vi "弹窗-设置周期.vi"() -> ()   [LabVIEW 2017]
panel:
  out "参考-单位":enum16{"年", "月", "日", "时", "分"}(ring)
  out "参考-定时模式":enum16{"绝对时间", "相对时间"}(ring)
  in  "超时":i32=1000
  out "目标时刻-导出":timestamp
  out "目标时刻-累积":timestamp
  out "定时器":T1
  in  "分别导出?":bool
  out "下个导出时刻":string
  in  "间隔-导出":u8=1 min=1 max=23
  in  "单位-导出":enum16{"年", "月", "日", "时", "分"}(ring)=enum."日"
  in  "定时模式-导出":enum16{"绝对时间", "相对时间"}(ring)
  out "提示语":string
  out "下个累积时刻":string caption="下个导出时刻"
  in  "间隔-累积":u8=1 min=1 max=59
  in  "单位-累积":enum16{"年", "月", "日", "时", "分"}(ring)=enum."日"
  in  "定时模式-累积":enum16{"绝对时间", "相对时间"}(ring)
  in  "确定":bool
  in  "取消":bool
  out "信号-关闭窗口":bool=TRUE
  # "累积周期"
  # "导出周期"
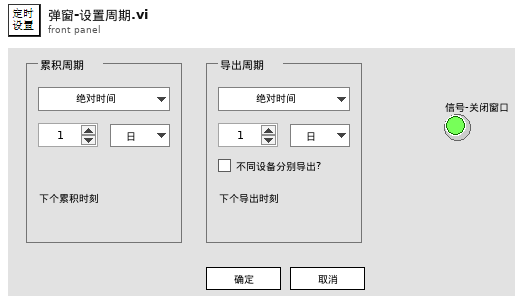
[diagram p1: front panel]
types:
  T1 = typedef "定时器枚举.ctl" = enum16{"累积定时", "导出定时"}
  T2 = typedef "定时配置.ctl" = cluster{"定时模式":enum16{"绝对时间", "相对时间"}, "单位":enum16{"年", "月", "日", "时", "分"}, "间隔":u8, "目标时刻":timestamp}
  T3 = enum32{"Invalid", "Standard", "Closed", "Hidden", "Minimized", "Maximized"}
  T4 = typedef "簇-输入.ctl" = cluster{"配置文件动作":T5, "数据输入":variant}
  T5 = typedef "枚举-配置文件动作.ctl" = enum16{"初始化加载配置", "读取配置", "写入-屏幕键盘", "写入-静音延迟", "写入-主要探头类型", "写入-串口配置", "写入-累积定时", "写入-导出定时", "保存配置到文件"}
  T6 = typedef "簇-定时配置.ctl" = cluster{"定时模式":enum16{"绝对时间", "相对时间"}, "单位":enum16{"年", "月", "日", "时", "分"}, "间隔":u8, "目标时刻":timestamp}
  T7 = typedef "簇-配置文件内容.ctl" = cluster{"调试模式？":bool, "屏幕键盘？":bool, "软件版本":string, "静音延迟 s":u16, "主要探头类型":T8, "串口配置":cluster{"COM口":refnum<visa-resource-name>, "波特率":enum16{"9600", "19200"}, "读写超时ms":i16, "丢包判定次数":i16}, "定时配置-累积分段":T6, "定时配置-自动导出":cluster{"定时配置-自动导出":T6, "分别导出?":bool}}
  T8 = typedef "枚举-主要探头类型.ctl" = enum16{"网络探头", "串口探头"}
  T9 = typedef "LVDateTimeRec.ctl" = cluster{"秒数的小数部分":dbl, "秒":i32, "分":i32, "时":i32, "日":i32, "月":i32, "年":i32, "天数（周）":i32, "天数（年）":i32, "DST":i32}
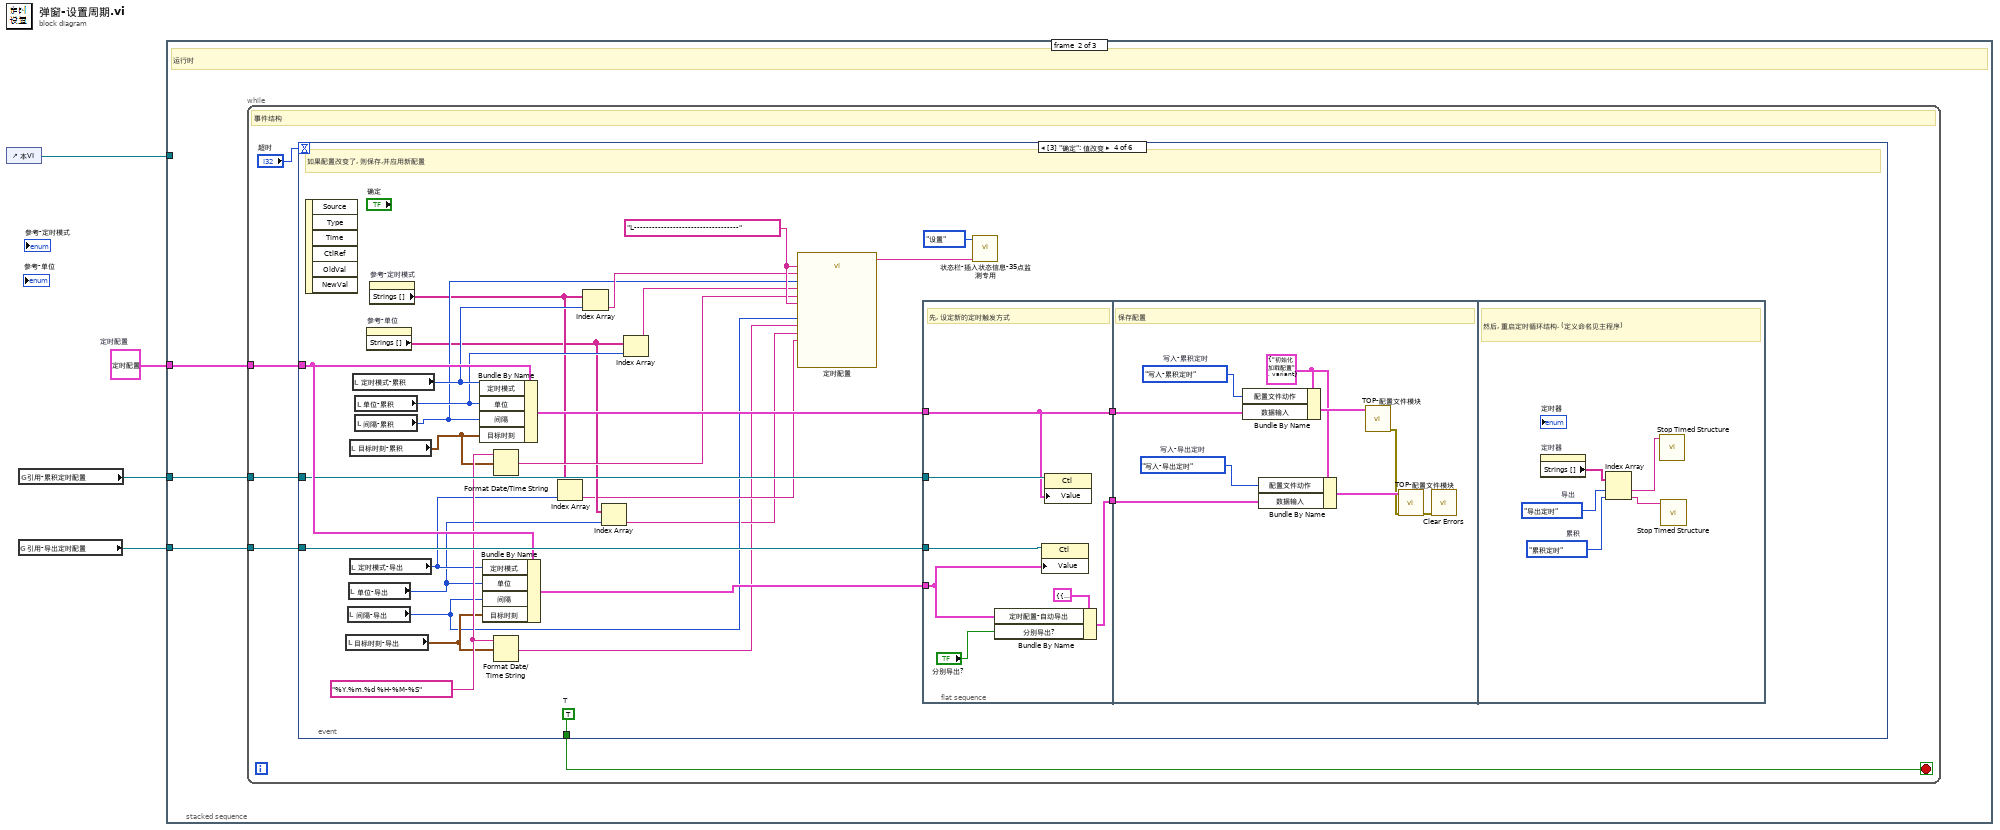
[diagram p0: block diagram]
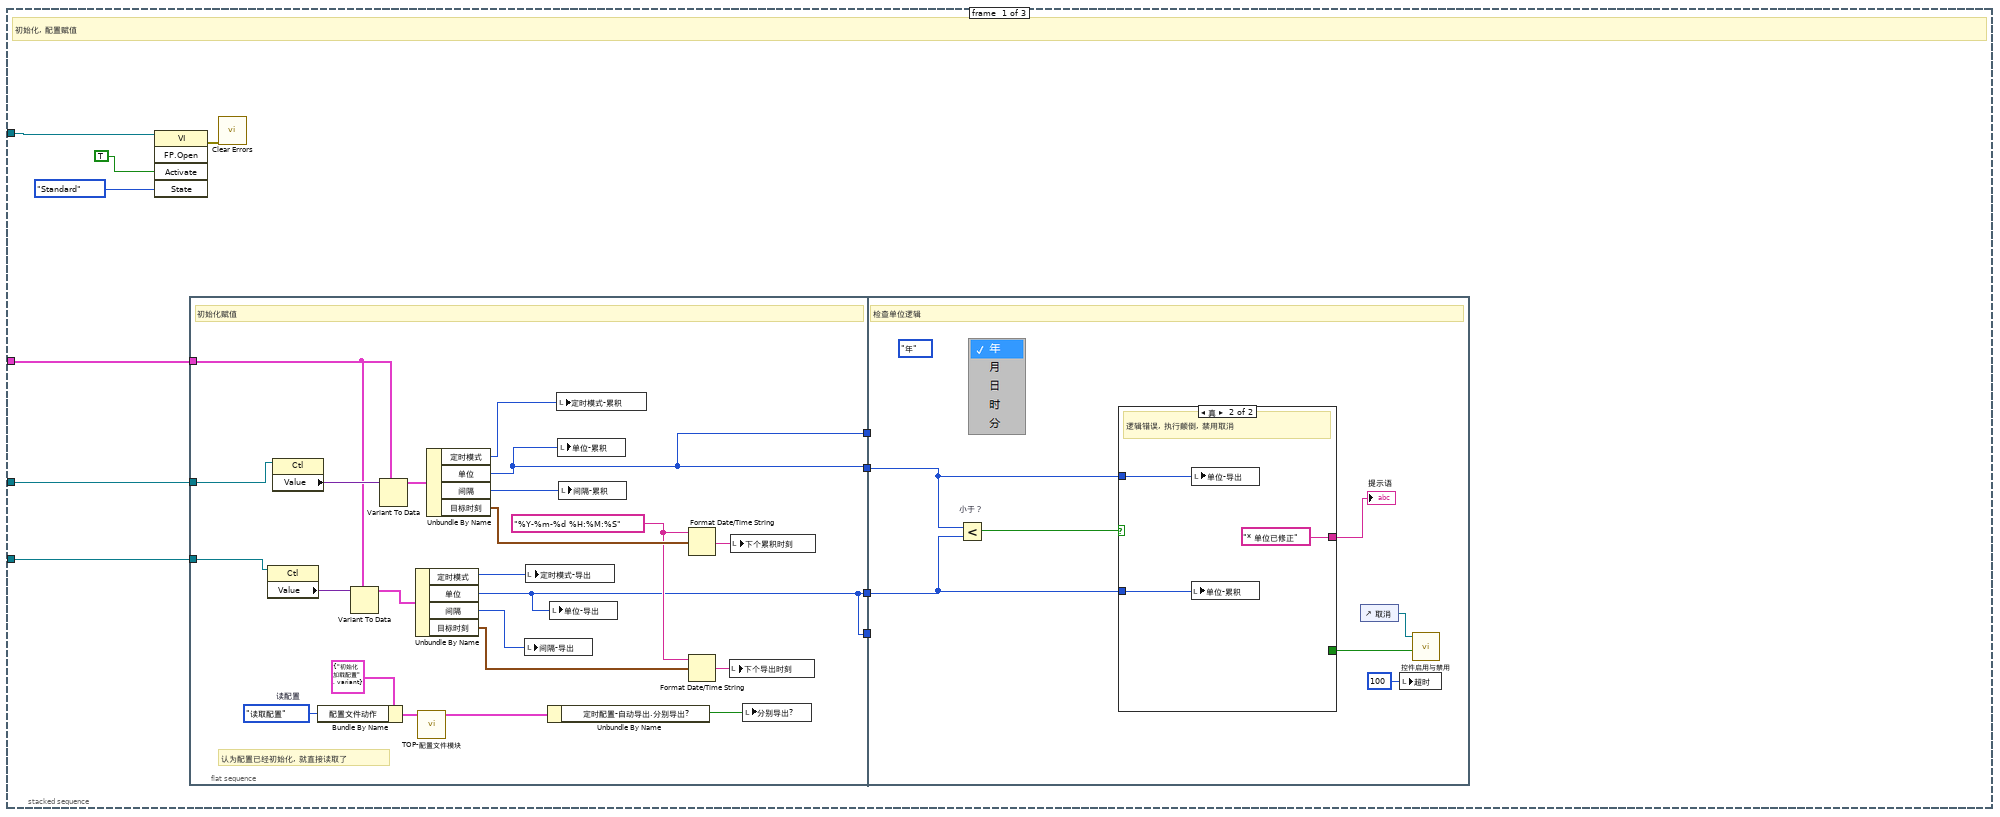
[diagram p2: hidden frame]
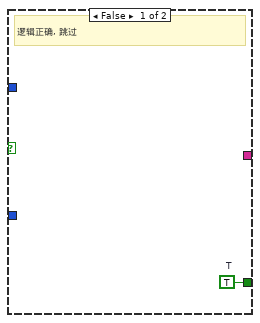
[diagram p3: hidden frame]
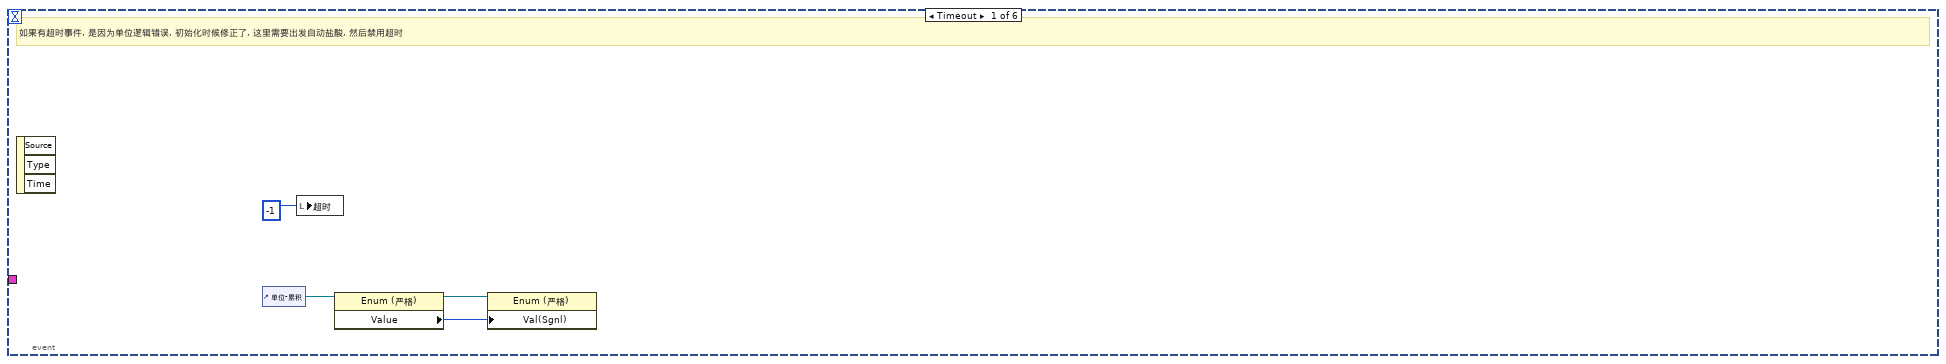
[diagram p4: hidden frame]
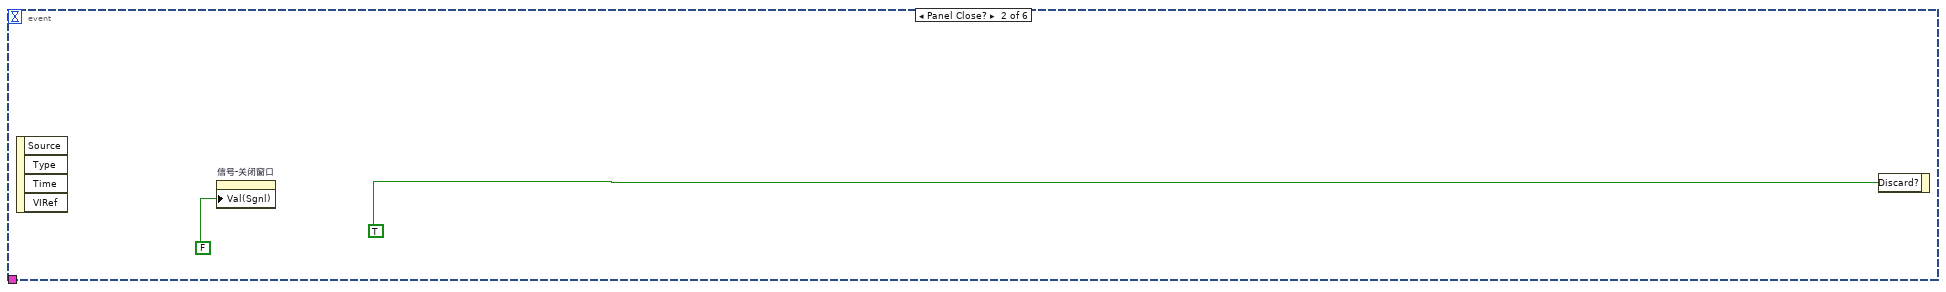
[diagram p5: hidden frame]
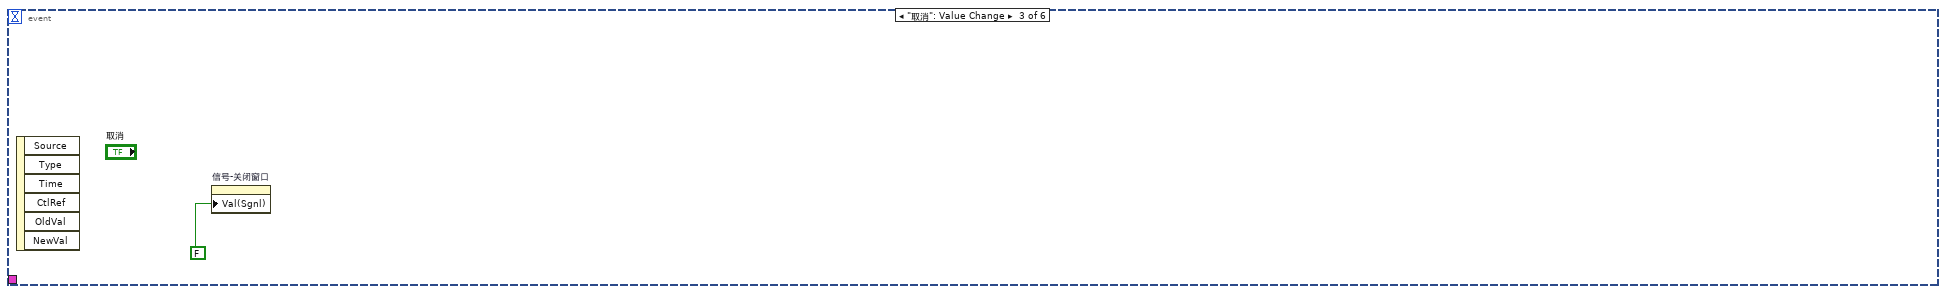
[diagram p6: hidden frame]
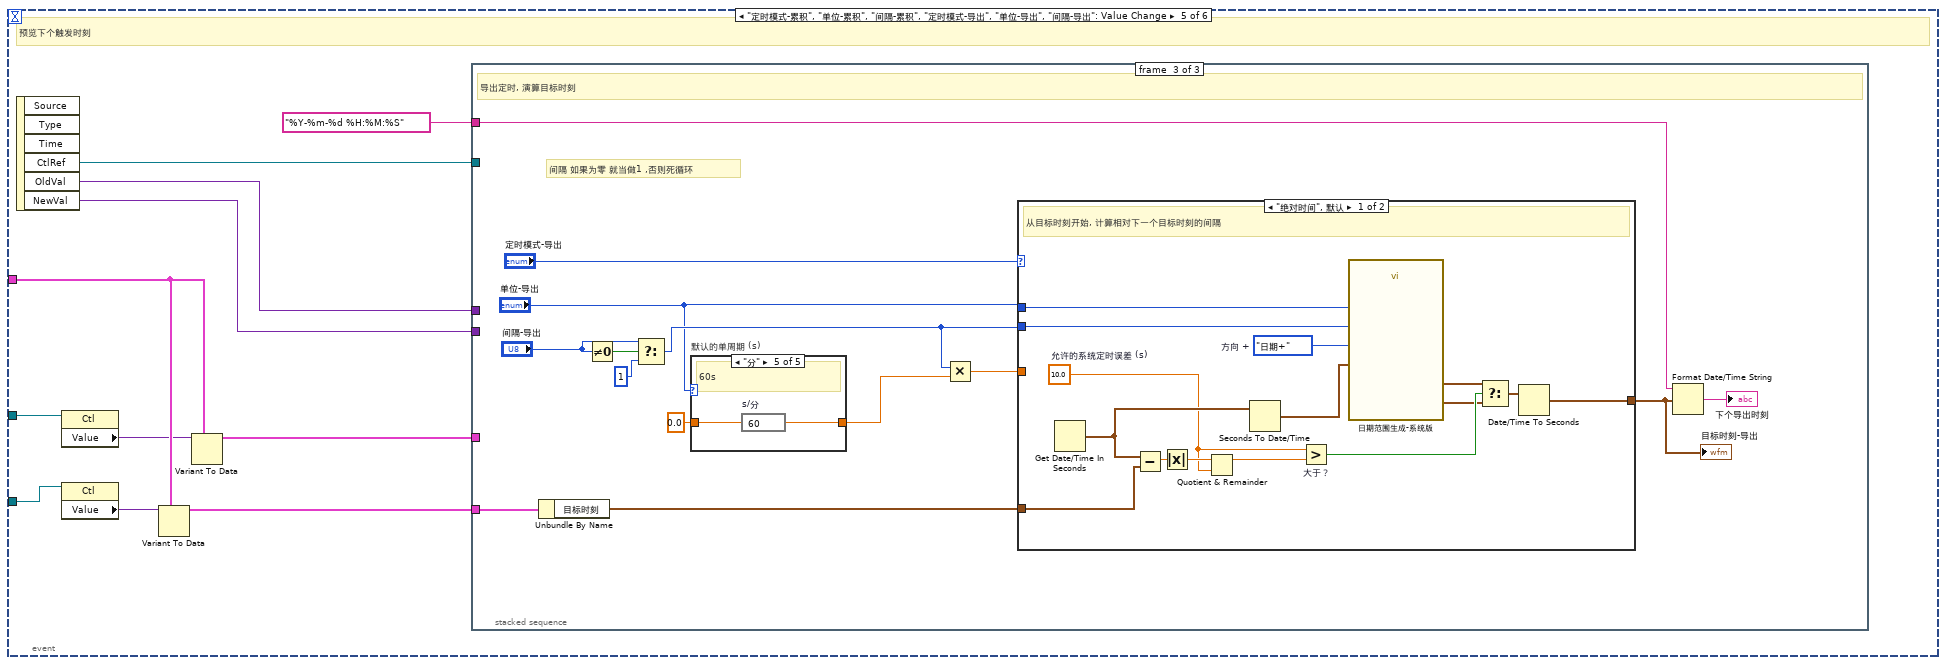
[diagram p7: hidden frame]
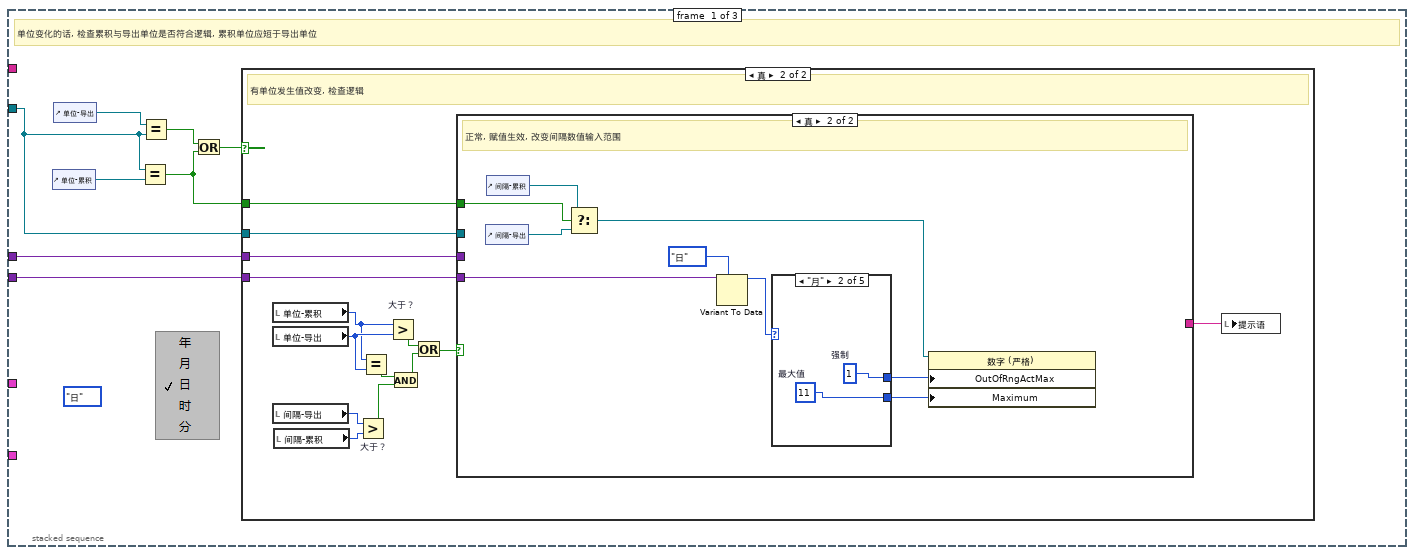
[diagram p8: hidden frame]
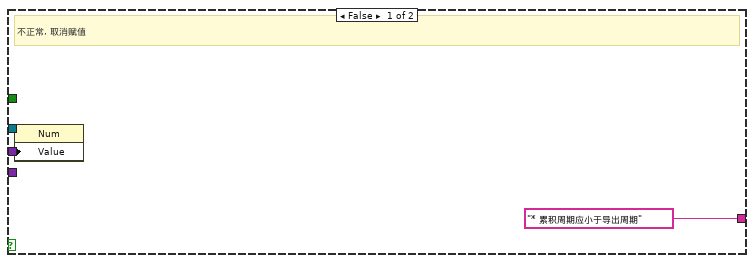
[diagram p10: hidden frame]
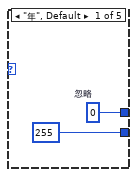
[diagram p11: hidden frame]
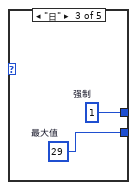
[diagram p12: hidden frame]
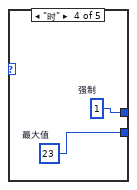
[diagram p13: hidden frame]
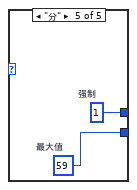
[diagram p14: hidden frame]
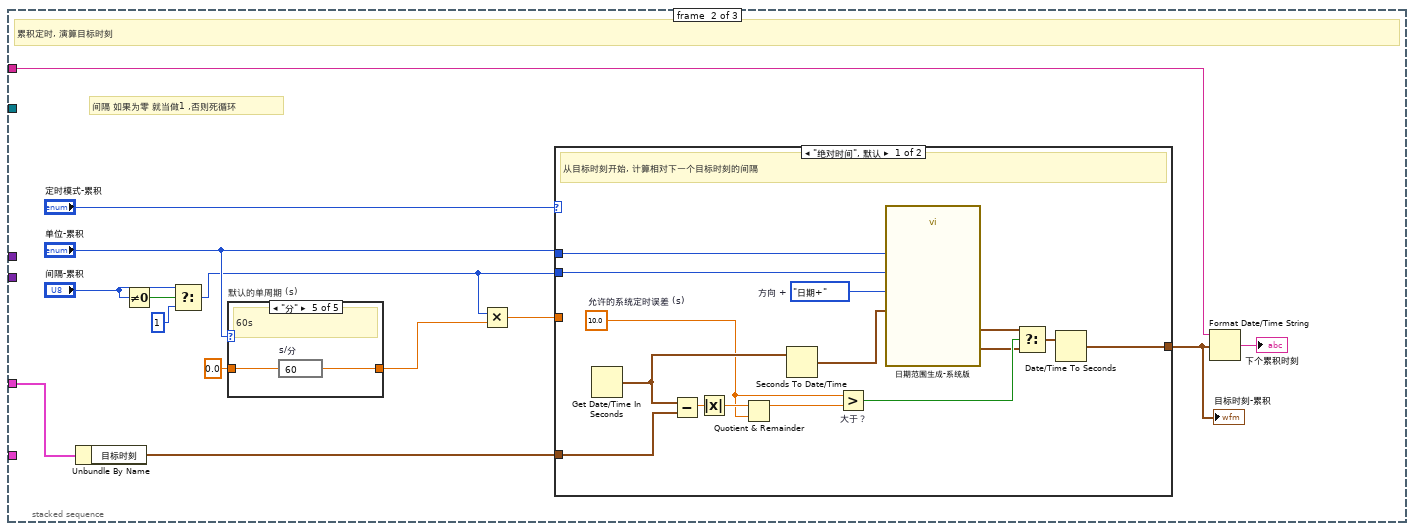
[diagram p15: hidden frame]
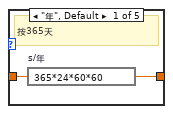
[diagram p16: hidden frame]
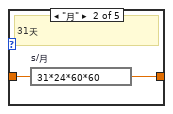
[diagram p17: hidden frame]
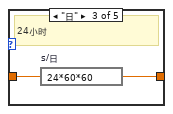
[diagram p18: hidden frame]
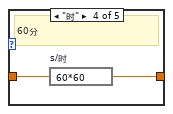
[diagram p19: hidden frame]
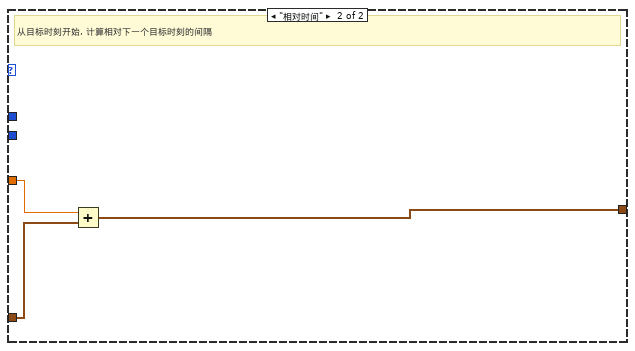
[diagram p20: hidden frame]
diagram:
  w3 = T2 {"定时模式"=enum."绝对时间", "单位"=enum."年", "间隔"=0, "目标时刻"=timestamp(0 s since 1904-01-01)}  # 定时配置
  n1 = control-ref of="本VI"() -> (w4:refnum<vi>)
  n2 = global read "全局变量-35点监测.vi" "引用-导出定时配置"() -> (w2:refnum<vi>)
  n3 = global read "全局变量-35点监测.vi" "引用-累积定时配置"() -> (w1:refnum<vi>)
  n4 = stacked-sequence {
    tunnel: w4 -> [w15 _ w257]
    tunnel: w2 -> [w11 w52 _]
    tunnel: w3 -> [w10 w51 _]
    tunnel: w1 -> [w12 w50 _]
    frame #0 {
      # "初始化, 配置赋值"
      n5 = invoke class="VI" method="FP.Open"(reference=w15, "Activate"=TRUE ("激活？"), "State"=T3."Standard" ("状态")) -> (error out=w9:errorcluster)  [unwired: 2 in, 4 out]
      n6 = flat-sequence {
        tunnel: w12 -> [w30]
        tunnel: w11 -> [w29]
        tunnel: w10 -> [w28]
        tunnel: [w21] -> w8
        tunnel: [w20] -> w7
        tunnel: [w21] -> w6
        tunnel: [w20] -> w5
        tunnel: w8 -> [w44]
        tunnel: w7 -> [w43]
        tunnel: w6 -> [_]
        tunnel: w5 -> [_]
        frame #0 {
          w16 = 枚举-配置文件动作."读取配置"  # 读配置
          w24 = "%Y-%m-%d %H:%M:%S" ("时间格式字符串(%c)")
          # "认为配置已经初始化, 就直接读取了"
          # "初始化赋值"
          n7 = property class="Ctl"(reference=w29) -> ("Value"=w32:variant)  [unwired: 1 in, 2 out]
          n8 = property class="Ctl"(reference=w30) -> ("Value"=w37:variant)  [unwired: 1 in, 2 out]
          n9 = Bundle By Name(cluster=T4 {"配置文件动作"=enum."初始化加载配置", "数据输入"=variant} ("输入"), "配置文件动作"=w16) -> (w17:T4)
          n10 = Variant To Data(type=w28, Variant=w32) -> (data=w31:T2)  [unwired: 1 in, 1 out]
          n11 = Variant To Data(type=w28, Variant=w37) -> (data=w38:T2)  [unwired: 1 in, 1 out]
          n12 = Unbundle By Name(w31) -> ("定时模式"=w26:enum16{"绝对时间", "相对时间"}, "单位"=w20:enum16{"年", "月", "日", "时", "分"}, "间隔"=w25:u8, "目标时刻"=w23:timestamp)
          n13 = call "TOP-配置文件模块.vi"("输入"=w17) -> ("配置文件"=w19:T7)  [unwired: 9 in, 1 out]
          n14 = Unbundle By Name(w38) -> ("定时模式"=w33:enum16{"绝对时间", "相对时间"}, "单位"=w21:enum16{"年", "月", "日", "时", "分"}, "间隔"=w34:u8, "目标时刻"=w36:timestamp)
          n15 = local write "间隔-导出"(w25) -> ()
          n16 = local write "定时模式-导出"(w26) -> ()
          n17 = Unbundle By Name(w19) -> ("定时配置-自动导出.分别导出?"=w27:bool)
          n18 = local write "单位-导出"(w20) -> ()
          n19 = local write "定时模式-累积"(w33) -> ()
          n20 = local write "单位-累积"(w21) -> ()
          n21 = local write "间隔-累积"(w34) -> ()
          n22 = Format Date/Time String(time format string (%c)=w24, seconds (now)=w36) -> (date/time string=w35:string)  [unwired: 1 in]
          n23 = Format Date/Time String(time format string (%c)=w24, seconds (now)=w23) -> (date/time string=w22:string)  [unwired: 1 in]
          n24 = local write "下个导出时刻"(w22) -> ()
          n25 = local write "下个累积时刻"(w35) -> ()
          n26 = local write "分别导出?"(w27) -> ()
        }
        frame #1 {
          (unwired) enum16{"年", "月", "日", "时", "分"}."年" ("单位")
          # "检查单位逻辑"
          n27 = Less? "小于？"(x=w44, y=w43) -> (x < y?=w45:bool)
          n28 = case shown="真" w45 {
            tunnel: w44 -> [_ w49]
            tunnel: w43 -> [_ w48]
            tunnel: [_ "* 单位已修正" ("提示语")] -> w40
            tunnel: [w46 _] -> w41
            frame False {
              w46 = TRUE  # T
              # "逻辑正确, 跳过"
            }
            frame True {
              # "逻辑错误, 执行颠倒, 禁用取消"
              n29 = local write "单位-累积"(w48) -> ()
              n30 = local write "单位-导出"(w49) -> ()
            }
          }
          "提示语" <- w40
          n31 = control-ref of="取消"() -> (w42:refnum<vi>)
          n32 = local write "超时"(100 ("超时")) -> ()
          n33 = call "控件启用与禁用.vi"("启用？"=w41, "控件引用"=w42) -> ()  [unwired: 9 in, 1 out]
        }
      }
      n34 = call <vilib>:"Clear Errors.vi"("error in (no error)"=w9) -> ()  [unwired: 5 in, 2 out]
    }
    frame #1 {
      # "运行时"
      n35 = while {
        tunnel: w52 -> [w56]
        tunnel: w51 -> [w55]
        tunnel: w50 -> [w54]
        stop <- w57 stop-if-true
        # "事件结构"
        n36 = event shown="[3] \"确定\": 值改变" {
          selector: _ -> [_ _ _ _ _ _]
          dyn-events: _ -> [_ _ _ _ _ _]
          timeout: "超时" -> [_ _ _ _ _ _]
          tunnel: [_ _ _ w92 _ TRUE] -> w57
          tunnel: w56 -> [_ _ _ w91 w123 _]
          tunnel: w55 -> [_ _ _ w88 w121 _]
          tunnel: w54 -> [_ _ _ w87 w122 _]
          event Timeout {
            # "如果有超时事件, 是因为单位逻辑错误, 初始化时候修正了, 这里需要出发自动盐酸, 然后禁用超时"
            n37 = event-data() -> ()  [unwired: 1 in, 3 out]
            n38 = control-ref of="单位-累积"() -> (w60:refnum<vi>)
            n39 = local write "超时"(-1 ("超时")) -> ()
            n40 = property class="Enum (严格)"(reference=w60) -> (reference out=w59:refnum<vi>, "Value"=w58:enum16{"年", "月", "日", "时", "分"})  [unwired: 1 in, 1 out]
            n41 = property class="Enum (严格)"(reference=w59, "Val(Sgnl)"=w58) -> ()  [unwired: 1 in, 2 out]
          }
          event Panel Close? {
            n42 = event-data() -> ()  [unwired: 1 in, 4 out]
            n43 = property on="信号-关闭窗口" class="Bool (严格)"("Val(Sgnl)"=FALSE ("值(信号)")) -> ()  [unwired: 2 in, 2 out]
            n44 = event-data("Discard?"=TRUE ("放弃？")) -> ()  [unwired: 1 in, 1 out]
          }
          event "取消": Value Change {
            n45 = event-data() -> ()  [unwired: 1 in, 6 out]
            n46 = property on="信号-关闭窗口" class="Bool (严格)"("Val(Sgnl)"=FALSE ("值(信号)")) -> ()  [unwired: 2 in, 2 out]
          }
          event "确定": Value Change {
            w80 = "%Y.%m.%d %H-%M-%S" ("时间格式字符串(%c)")
            w77 = "L-----------------------------------" ("字符串")
            w92 = TRUE  # T
            # "如果配置改变了, 则保存,并应用新配置"
            n47 = event-data() -> ()  [unwired: 1 in, 6 out]
            n48 = local read "目标时刻-导出"() -> (w79:timestamp)
            n49 = local read "间隔-导出"() -> (w67:u8)
            n50 = local read "单位-导出"() -> (w69:enum16{"年", "月", "日", "时", "分"})
            n51 = local read "目标时刻-累积"() -> (w78:timestamp)
            n52 = local read "定时模式-导出"() -> (w70:enum16{"绝对时间", "相对时间"})
            n53 = local read "定时模式-累积"() -> (w83:enum16{"绝对时间", "相对时间"})
            n54 = local read "单位-累积"() -> (w81:enum16{"年", "月", "日", "时", "分"})
            n55 = local read "间隔-累积"() -> (w75:u8)
            n56 = property on="参考-单位" class="Enum (严格)"() -> ("Strings []"=w71:string[])  [unwired: 2 in, 2 out]
            n57 = property on="参考-定时模式" class="Enum (严格)"() -> ("Strings []"=w72:string[])  [unwired: 2 in, 2 out]
            n58 = Bundle By Name(cluster=w88, "定时模式"=w83, "单位"=w81, "间隔"=w75, "目标时刻"=w78) -> (w90:T2)
            n59 = Bundle By Name(cluster=w88, "定时模式"=w70, "单位"=w69, "间隔"=w67, "目标时刻"=w79) -> (w86:T2)
            n60 = Format Date/Time String(time format string (%c)=w80, seconds (now)=w78) -> (date/time string=w73:string)  [unwired: 1 in]
            n61 = Format Date/Time String(time format string (%c)=w80, seconds (now)=w79) -> (date/time string=w65:string)  [unwired: 1 in]
            n62 = Index Array(array=w72, index=w70) -> (element=w68:string)
            n63 = Index Array(array=w72, index=w83) -> (element=w76:string)
            n64 = Index Array(array=w71, index=w69) -> (element=w66:string)
            n65 = Index Array(array=w71, index=w81) -> (element=w74:string)
            n66 = call "定时配置"("补充_累"=w77, "模式_累"=w76, "间隔_累"=w75, "周期_类"=w74, "下个_累"=w73, "补充_导"=w77, "模式_导"=w68, "间隔_导"=w67, "周期_导"=w66, "下个_导"=w65) -> ("Result"=w82:string)  [unwired: 16 in, 1 out]
            n67 = flat-sequence {
              tunnel: [w97] -> w89
              tunnel: w90 -> [w97]
              tunnel: w91 -> [w99]
              tunnel: w87 -> [w98]
              tunnel: w86 -> [w95]
              tunnel: [w93] -> w85
              tunnel: w89 -> [w102]
              tunnel: w85 -> [w101]
              frame #0 {
                # "先, 设定新的定时触发方式"
                n68 = Bundle By Name(cluster=cluster{"定时配置-自动导出":T6, "分别导出?":bool} {"定时配置-自动导出"={"定时模式"=enum."绝对时间", "单位"=enum."年", "间隔"=0, "目标时刻"=timestamp(0 s since 1904-01-01)}, "分别导出?"=FALSE} ("定时配置-自动导出"), "定时配置-自动导出"=w95, "分别导出?"="分别导出?") -> (w93:cluster{"定时配置-自动导出":T6, "分别导出?":bool})
                n69 = property class="Ctl"(reference=w99, "Value"=w95) -> ()  [unwired: 1 in, 2 out]
                n70 = property class="Ctl"(reference=w98, "Value"=w97) -> ()  [unwired: 1 in, 2 out]
              }
              frame #1 {
                w105 = 枚举-配置文件动作."写入-导出定时"  # 写入-导出定时
                w106 = 枚举-配置文件动作."写入-累积定时"  # 写入-累积定时
                w104 = T4 {"配置文件动作"=enum."初始化加载配置", "数据输入"=variant} ("输入")
                # "保存配置"
                n71 = Bundle By Name(cluster=w104, "配置文件动作"=w106, "数据输入"=w102) -> (w107:T4)
                n72 = Bundle By Name(cluster=w104, "配置文件动作"=w105, "数据输入"=w101) -> (w108:T4)
                n73 = call "TOP-配置文件模块.vi"("输入"=w107) -> ("error out"=w103:errorcluster)  [unwired: 9 in, 1 out]
                n74 = call "TOP-配置文件模块.vi"("error in (no error)"=w103, "输入"=w108) -> ("error out"=w100:errorcluster)  [unwired: 8 in, 1 out]
                n75 = call <vilib>:"Clear Errors.vi"("error in (no error)"=w100) -> ()  [unwired: 5 in, 2 out]
              }
              frame #2 {
                w109 = 定时器枚举."累积定时"  # 累积
                w110 = 定时器枚举."导出定时"  # 导出
                # "然后, 重启定时循环结构. (定义命名见主程序)"
                n76 = property on="定时器" class="Enum (严格)"() -> ("Strings []"=w113:string[])  [unwired: 2 in, 2 out]
                n77 = Index Array(array=w113, index #1=w110, index #2=w109) -> (element #1=w112:string, element #2=w111:string)
                n78 = call <vilib>:"Stop Timed Structure.vi"("name"=w112) -> ()  [unwired: 10 in, 1 out]
                n79 = call <vilib>:"Stop Timed Structure.vi"("name"=w111) -> ()  [unwired: 10 in, 1 out]
              }
            }
            n80 = call "状态栏-插入状态信息-35点监测专用.vi"("消息内容"=w82, "状态类型"=enum16{"全部", "报警", "通信", "设置"}."设置") -> ()  [unwired: 10 in]
          }
          event "定时模式-累积", "单位-累积", "间隔-累积", "定时模式-导出", "单位-导出", "间隔-导出": Value Change {
            # "预览下个触发时刻"
            n81 = event-data() -> ("CtlRef"=w119:refnum<vi>, "OldVal"=w116:variant, "NewVal"=w115:variant)  [unwired: 1 in, 3 out]
            n82 = property class="Ctl"(reference=w122) -> ("Value"=w120:variant)  [unwired: 1 in, 2 out]
            n83 = property class="Ctl"(reference=w123) -> ("Value"=w124:variant)  [unwired: 1 in, 2 out]
            n84 = Variant To Data(type=w121, Variant=w124) -> (data=w117:T2)  [unwired: 1 in, 1 out]
            n85 = Variant To Data(type=w121, Variant=w120) -> (data=w118:T2)  [unwired: 1 in, 1 out]
            n86 = stacked-sequence {
              tunnel: w119 -> [w128 _ _]
              tunnel: w118 -> [_ w169 _]
              tunnel: w117 -> [_ _ w218]
              tunnel: w116 -> [w129 _ _]
              tunnel: w115 -> [w125 _ _]
              tunnel: "%Y-%m-%d %H:%M:%S" ("时间格式字符串(%c)") -> [_ w171 w216]
              frame #0 {
                (unwired) enum16{"年", "月", "日", "时", "分"}."日" ("单位-累积")
                # "单位变化的话, 检查累积与导出单位是否符合逻辑, 累积单位应短于导出单位"
                n87 = control-ref of="单位-累积"() -> (w130:refnum<vi>)
                n88 = control-ref of="单位-导出"() -> (w131:refnum<vi>)
                n89 = Equal?(x=w128, y=w130) -> (x = y?=w126:bool)
                n90 = Equal?(x=w131, y=w128) -> (x = y?=w132:bool)
                n91 = Or(x=w132, y=w126) -> (x .or. y?=w127:bool)
                n92 = case shown="真" w127 {
                  tunnel: w129 -> [_ w144]
                  tunnel: w128 -> [_ w145]
                  tunnel: w126 -> [_ w143]
                  tunnel: w125 -> [_ w142]
                  frame False {
                    # "没有单位变化"
                  }
                  frame True {
                    # "有单位发生值改变, 检查逻辑"
                    n93 = local read "单位-累积"() -> (w138:enum16{"年", "月", "日", "时", "分"})
                    n94 = local read "单位-导出"() -> (w139:enum16{"年", "月", "日", "时", "分"})
                    n95 = local read "间隔-导出"() -> (w136:u8)
                    n96 = local read "间隔-累积"() -> (w135:u8)
                    n97 = Greater? "大于？"(x=w136, y=w135) -> (0:w134:bool)
                    n98 = Equal?(x=w138, y=w139) -> (x = y?=w137:bool)
                    n99 = Greater? "大于？"(x=w138, y=w139) -> (0:w146:bool)
                    n100 = And(x=w137, y=w134) -> (x .and. y?=w133:bool)
                    n101 = Or(x=w146, y=w133) -> (x .or. y?=w140:bool)
                    n102 = case shown="真" w140 {
                      tunnel: w145 -> [w149 _]
                      tunnel: w144 -> [w148 _]
                      tunnel: w143 -> [_ w155]
                      tunnel: w142 -> [_ w151]
                      tunnel: ["* 累积周期应小于导出周期" ("提示语") _] -> w141
                      frame False {
                        # "不正常, 取消赋值"
                        n103 = property class="Num"(reference=w149, "Value"=w148) -> ()  [unwired: 1 in, 2 out]
                      }
                      frame True {
                        # "正常, 赋值生效, 改变间隔数值输入范围"
                        n104 = control-ref of="间隔-导出"() -> (w154:refnum<vi>)
                        n105 = control-ref of="间隔-累积"() -> (w153:refnum<vi>)
                        n106 = Select(t=w153, s=w155, f=w154) -> (s? t:f=w152:refnum<vi>)
                        n107 = Variant To Data(type=enum16{"年", "月", "日", "时", "分"}."日" ("单位-累积"), Variant=w151) -> (data=w158:enum16{"年", "月", "日", "时", "分"})  [unwired: 1 in, 1 out]
                        n108 = case shown="\"月\"" w158 {
                          tunnel: [w160 w162 w164 w166 w168] -> w157
                          tunnel: [u8 255 w161 w163 w165 w167] -> w156
                          frame "年", Default {
                            w160 = u8 0  # 忽略
                          }
                          frame "月" {
                            w161 = u8 11  # 最大值
                            w162 = u8 1  # 强制
                          }
                          frame "日" {
                            w163 = u8 29  # 最大值
                            w164 = u8 1  # 强制
                          }
                          frame "时" {
                            w165 = u8 23  # 最大值
                            w166 = u8 1  # 强制
                          }
                          frame "分" {
                            w167 = u8 59  # 最大值
                            w168 = u8 1  # 强制
                          }
                        }
                        n109 = property on="属性节点" class="数字 (严格)"(reference=w152, "OutOfRngActMax"=w157, "Maximum"=w156) -> ()  [unwired: 1 in, 2 out]
                      }
                    }
                    n110 = local write "提示语"(w141) -> ()
                  }
                }
              }
              frame #1 {
                # "间隔 如果为零 就当做1 ,否则死循环"
                # "累积定时, 演算目标时刻"
                n111 = Unbundle By Name(w169) -> ("目标时刻"=w172:timestamp)
                n112 = Not Equal To 0?(x="间隔-累积") -> (x != 0?=w177:bool)
                n113 = Select(t="间隔-累积", s=w177, f=u8 1 ("间隔")) -> (s? t:f=w176:u8)
                n114 = case "默认的单周期 (s)" shown="\"分\"" "单位-累积" {
                  tunnel: [w184 w186 w188 w190 w192] -> w179
                  tunnel: 0.0 -> [w183 w185 w187 w189 w191]
                  frame "年", Default {
                    # "按365天"
                    n115 = expression code="365*24*60*60" "s/年"(w183) -> (w184:dbl)
                  }
                  frame "月" {
                    # "31天"
                    n116 = expression code="31*24*60*60" "s/月"(w185) -> (w186:dbl)
                  }
                  frame "日" {
                    # "24小时"
                    n117 = expression code="24*60*60" "s/日"(w187) -> (w188:dbl)
                  }
                  frame "时" {
                    # "60分"
                    n118 = expression code="60*60" "s/时"(w189) -> (w190:dbl)
                  }
                  frame "分" {
                    # "60s"
                    n119 = expression code="60" "s/分"(w191) -> (w192:dbl)
                  }
                }
                n120 = Multiply(x=w176, y=w179) -> (x*y=w178:dbl)
                n121 = case shown="\"绝对时间\", 默认" "定时模式-累积" {
                  tunnel: "单位-累积" -> [w207 _]
                  tunnel: w176 -> [w202 _]
                  tunnel: w172 -> [w203 w209]
                  tunnel: w178 -> [_ w210]
                  tunnel: [w201 w208] -> w170
                  frame "绝对时间", Default {
                    w193 = 10.0  # 允许的系统定时误差 (s)
                    w200 = enum16{"当前", "日期+", "日期-"}."日期+"  # 方向 +
                    # "从目标时刻开始, 计算相对下一个目标时刻的间隔"
                    n122 = Get Date/Time In Seconds() -> (seconds since 1Jan1904=w204:timestamp)
                    n123 = Subtract(x=w204, y=w203) -> (x-y=w205:dbl)
                    n124 = Absolute Value(x=w205) -> (abs(x)=w195:dbl)
                    n125 = Quotient & Remainder(x=w195, y=w193) -> (x-y*floor(x/y)=w194:dbl)  [unwired: 1 out]
                    n126 = Seconds To Date/Time(time stamp (now)=w204) -> (date time rec=w206:T9)  [unwired: 1 in]
                    n127 = Greater? "大于？"(x=w193, y=w194) -> (0:w199:bool)
                    n128 = call "日期范围生成-系统版.vi"("单位"=w207, "方向"=w200, "变化量(1)"=w202, "日期时间记录"=w206) -> ("下限"=w197:T9, "上限"=w196:T9)  [unwired: 6 in]
                    n129 = Select(t=w197, s=w199, f=w196) -> (s? t:f=w198:T9)
                    n130 = Date/Time To Seconds(2:w198) -> (0:w201:timestamp)  [unwired: 1 in]
                  }
                  frame "相对时间" {
                    # "从目标时刻开始, 计算相对下一个目标时刻的间隔"
                    n131 = Add(x=w210, y=w209) -> (x+y=w208:timestamp)
                  }
                }
                "目标时刻-累积" <- w170
                n132 = Format Date/Time String(time format string (%c)=w171, seconds (now)=w170) -> (date/time string=→"下个累积时刻":string)  [unwired: 1 in]
              }
              frame #2 {
                # "间隔 如果为零 就当做1 ,否则死循环"
                # "导出定时, 演算目标时刻"
                n133 = Unbundle By Name(w218) -> ("目标时刻"=w217:timestamp)
                n134 = Not Equal To 0?(x="间隔-导出") -> (x != 0?=w222:bool)
                n135 = Select(t="间隔-导出", s=w222, f=u8 1 ("间隔")) -> (s? t:f=w221:u8)
                n136 = case "默认的单周期 (s)" shown="\"分\"" "单位-导出" {
                  tunnel: [w226 w228 w230 w232 w234] -> w224
                  tunnel: 0.0 -> [w225 w227 w229 w231 w233]
                  frame "年", Default {
                    # "按365天"
                    n137 = expression code="365*24*60*60" "s/年"(w225) -> (w226:dbl)
                  }
                  frame "月" {
                    # "31天"
                    n138 = expression code="31*24*60*60" "s/月"(w227) -> (w228:dbl)
                  }
                  frame "日" {
                    # "24小时"
                    n139 = expression code="24*60*60" "s/日"(w229) -> (w230:dbl)
                  }
                  frame "时" {
                    # "60分"
                    n140 = expression code="60*60" "s/时"(w231) -> (w232:dbl)
                  }
                  frame "分" {
                    # "60s"
                    n141 = expression code="60" "s/分"(w233) -> (w234:dbl)
                  }
                }
                n142 = Multiply(x=w221, y=w224) -> (x*y=w223:dbl)
                n143 = case shown="\"绝对时间\", 默认" "定时模式-导出" {
                  tunnel: "单位-导出" -> [w249 _]
                  tunnel: w221 -> [w244 _]
                  tunnel: w217 -> [w245 w251]
                  tunnel: w223 -> [_ w252]
                  tunnel: [w243 w250] -> w212
                  frame "绝对时间", Default {
                    w235 = 10.0  # 允许的系统定时误差 (s)
                    w242 = enum16{"当前", "日期+", "日期-"}."日期+"  # 方向 +
                    # "从目标时刻开始, 计算相对下一个目标时刻的间隔"
                    n144 = Get Date/Time In Seconds() -> (seconds since 1Jan1904=w246:timestamp)
                    n145 = Subtract(x=w246, y=w245) -> (x-y=w247:dbl)
                    n146 = Absolute Value(x=w247) -> (abs(x)=w237:dbl)
                    n147 = Quotient & Remainder(x=w237, y=w235) -> (x-y*floor(x/y)=w236:dbl)  [unwired: 1 out]
                    n148 = Seconds To Date/Time(time stamp (now)=w246) -> (date time rec=w248:T9)  [unwired: 1 in]
                    n149 = Greater? "大于？"(x=w235, y=w236) -> (0:w241:bool)
                    n150 = call "日期范围生成-系统版.vi"("单位"=w249, "方向"=w242, "变化量(1)"=w244, "日期时间记录"=w248) -> ("下限"=w239:T9, "上限"=w238:T9)  [unwired: 6 in]
                    n151 = Select(t=w239, s=w241, f=w238) -> (s? t:f=w240:T9)
                    n152 = Date/Time To Seconds(2:w240) -> (0:w243:timestamp)  [unwired: 1 in]
                  }
                  frame "相对时间" {
                    # "从目标时刻开始, 计算相对下一个目标时刻的间隔"
                    n153 = Add(x=w252, y=w251) -> (x+y=w250:timestamp)
                  }
                }
                "目标时刻-导出" <- w212
                n154 = Format Date/Time String(time format string (%c)=w216, seconds (now)=w212) -> (date/time string=→"下个导出时刻":string)  [unwired: 1 in]
              }
            }
          }
          event "信号-关闭窗口": Value Change {
            # "关闭窗口, 询问?"
            n155 = event-data() -> ()  [unwired: 1 in, 6 out]
          }
        }
      }
    }
    frame #2 {
      # "结束"
      n156 = invoke class="VI" method="FP.Close"(reference=w257) -> (reference out=w256:refnum<vi>, error out=w255:errorcluster)  [unwired: 2 in, 1 out]
      n157 = invoke class="VI" method="Abort VI"(reference=w256, error in=w255) -> (error out=w254:errorcluster)  [unwired: 1 in, 2 out]
      n158 = call <vilib>:"Clear Errors.vi"("error in (no error)"=w254) -> ()  [unwired: 5 in, 2 out]
    }
  }
